vi "Two 8-bit Port Digital Input.vi"(2 "Two 8-bit DI Ports":T1={"8-bit DI Port 0"="Chassis1/Mod4/DI7:0", "8-bit DI Port 1"="Chassis1/Mod4/DI7:0"}) -> (7 "Packet":u64)   [LabVIEW 2010]
uses:
  <vilib>/eio/EIONode/EIONode.xnode
  <vilib>/rvi/eio/nirviEIOImplementation/nirviEIOImplementation.xnode
  <vilib>/rvi/eio/common/nirviEmuClasses.ctl
  <vilib>/rvi/eio/common/nirviEmuTemplateMethod_noerrors.vi
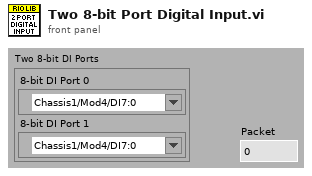
[diagram p1: front panel]
types:
  T1 = cluster{"8-bit DI Port 0":refnum<k21>, "8-bit DI Port 1":refnum<k21>}
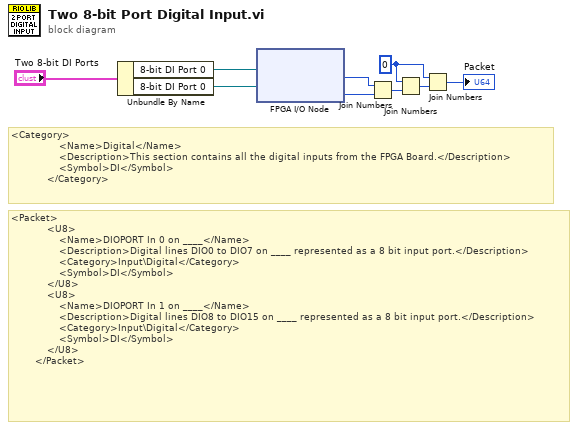
[diagram p0: block diagram]
diagram:
  w7 = u8 0 ("hi")
  # "<Packet>\n            <U8>\n                <Name>DIOPORT In 0 on ____</Name>\n                <Description>Digital lines DIO0 to DIO7 on ____ represented as a 8 bit input port.</Description>\n                <Category>Input\\Digital</Category>\n                <Symbol>DI</Symbol>\n            </U8>\n            <U8>\n                <Name>DIOPORT In 1 on ____</Name>\n                <Description>Digital lines DIO8 to DIO15 on ____ represented as a 8 bit input port.</Description>\n                <Category>Input\\Digital</Category>\n                <Symbol>DI</Symbol>\n            </U8>\n        </Packet>"
  # "<Category>\n                <Name>Digital</Name>\n                <Description>This section contains all the digital inputs from the FPGA Board.</Description>\n                <Symbol>DI</Symbol>\n            </Category>"
  n1 = Unbundle By Name("Two 8-bit DI Ports") -> ("8-bit DI Port 0"=w2:refnum<k21>, "8-bit DI Port 0"=w3:refnum<k21>)
  n2 = xnode "FPGA I/O Node"("FPGA I/O In"=w2, "FPGA I/O In"=w3) -> ("I/O Item"=w1:u8, "I/O Item"=w6:u8)  [unwired: 2 out]
  n3 = Join Numbers(hi=w1, lo=w6) -> ((hi.lo)=w9:u16)
  n4 = Join Numbers(hi=w7, lo=w9) -> ((hi.lo)=w8:u32)
  n5 = Join Numbers(hi=w7, lo=w8) -> ((hi.lo)=→"Packet":u64)
